vi "RetrievePix.vi"(11 "RawDataFile":path) -> ()   [LabVIEW 2015]
panel:
  out "Array":picture[](array[picture])
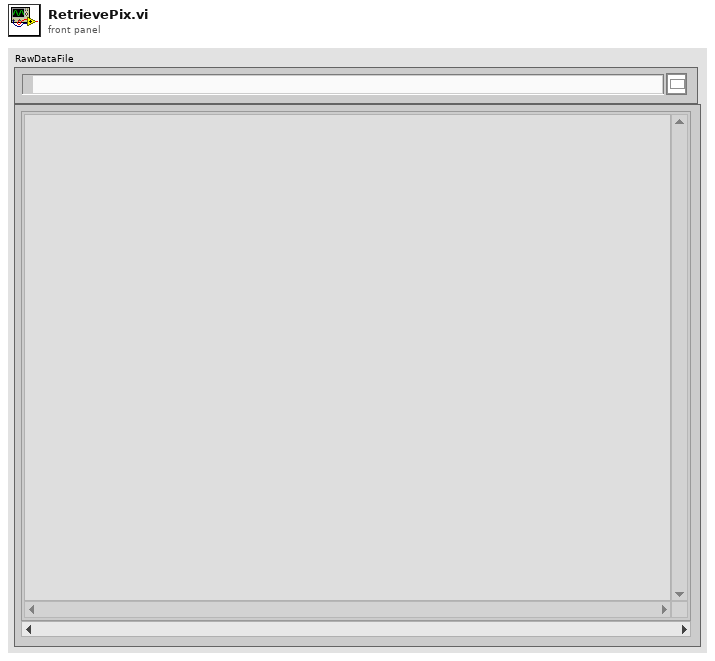
[diagram p1: front panel]
types:
  T1 = typedef "imagedata.ctl" = cluster{"image type":i32, "image depth":i32, "image":u8[], "mask":u8[], "colors":u32[], "Rectangle":cluster{"left":i16, "top":i16, "right":i16, "bottom":i16}}
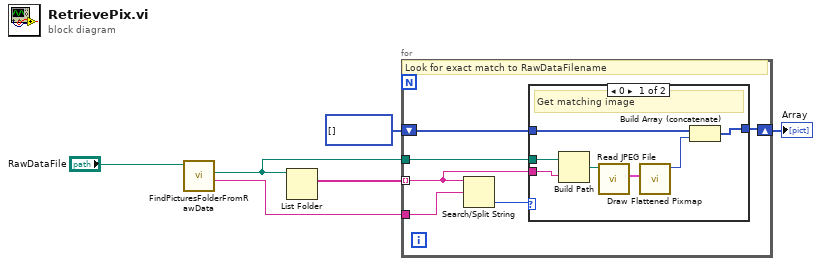
[diagram p0: block diagram]
diagram:
  n1 = call "FindPicturesFolderFromRawData.vi"("RawDataFile"="RawDataFile") -> ("RawDataName"=w4:string, "PicturesPath"=w3:path)  [unwired: 9 in]
  n2 = List Folder(path=w3) -> (filenames=w5:string[])  [unwired: 3 in, 3 out]
  n3 = for {
    tunnel: w5 -> [w7] mode=indexing
    tunnel: w4 -> [w12]
    shift-right: [w9] -> w2
    shift-left: picture[] [] -> [w10]
    tunnel: w3 -> [w8]
    # "Look for exact match to RawDataFilename"
    n4 = Search/Split String(string=w7, search string/char (-)=w12) -> (offset of match=w11:i32)  [unwired: 1 in, 2 out]
    n5 = case shown="0" w11 {
      tunnel: w10 -> [w19 w20]
      tunnel: [w18 w20] -> w9
      tunnel: w8 -> [w17 _]
      tunnel: w7 -> [w13 _]
      frame 0 {
        # "Get matching image"
        n6 = Build Path(base path=w17, name or relative path=w13) -> (appended path=w15:path)
        n7 = call <vilib>:"Read JPEG File.vi"("path to JPEG file"=w15) -> ("image data"=w16:T1)  [unwired: 8 in, 2 out]
        n8 = call <vilib>:"Draw Flattened Pixmap.vi"("image data"=w16) -> ("new picture"=w14:picture)  [unwired: 8 in]
        n9 = Build Array (concatenate)(w19, w14) -> (w18:picture[])
      }
      frame -1, Default {
        # "Not found"
      }
    }
  }
  "Array" <- w2
